vi "Multimode.vi"(2 "intervals":i32=100, 3 "X":dbl[](array[numeric]) format="%0.2f") -> (0 "error":i32, 1 "Modes":dbl[](array[numeric]) format="%0.2f")   [LabVIEW 2017, in "NI_AALBase.lvlib"]
doc: "Finds the modes (most common values) or estimated modes (most common range centers) of the input sequence <B>X</B>. This VI can perform unimodal or multimodal analysis. You must manually select the polymorphic instance to use."
uses:
  NI_AALBase.lvlib
  lvanlys.dll
panel:
  # "Multimode"
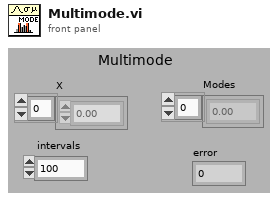
[diagram p1: front panel]
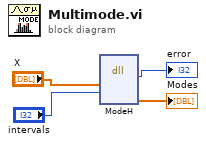
[diagram p0: block diagram]
diagram:
  n1 = dll-call lib="C:/Program Files/National Instruments/LabVIEW 2017/resource/lvanlys.*" fn="ModeH"("X"="X", "intervals"="intervals") -> (→"error":i32, "Modes"=→"Modes":dbl[])  [unwired: 6 in, 2 out]
